vi "Rcv Caller Notice.vi"(7 "Actor Name":string, 8 "error in (no error)":errorcluster, 9 "Params":variant, 10 "Action Name":string, 11 "Generic Actor in":refnum<class "Generic Actor.lvclass">) -> (0 "error out":errorcluster, 3 "Generic Actor out":refnum<class "Generic Actor.lvclass">)   [LabVIEW 2020, in "Generic Actor.lvlib" / "Generic Actor.lvclass"]
uses:
  Generic Actor.lvclass
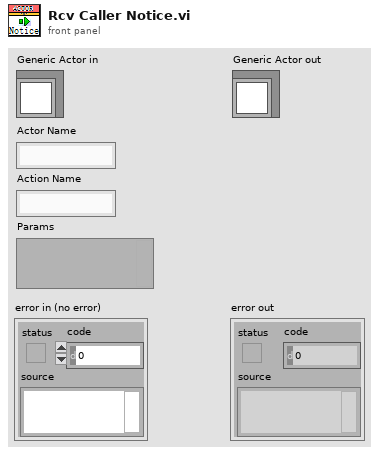
[diagram p1: front panel]
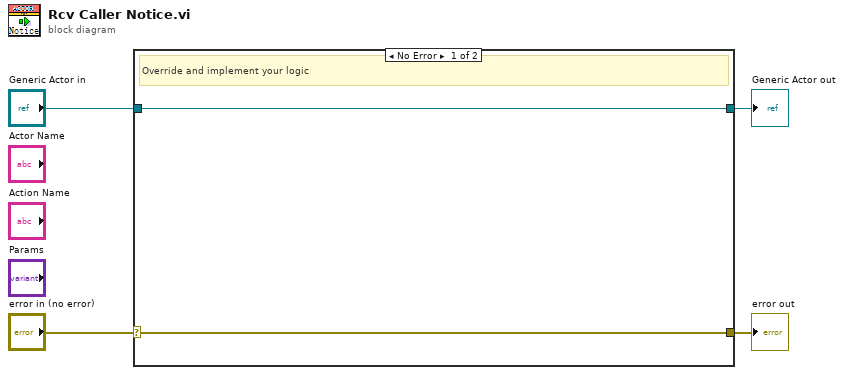
[diagram p0: block diagram]
diagram:
  n1 = case shown="No Error" "error in (no error)" {
    selector: "error in (no error)" -> [w5 w8]
    tunnel: [w5 w8] -> w3
    tunnel: [w6 w7] -> w1
    tunnel: "Generic Actor in" -> [w6 w7]
    frame No Error {
      # "Override and implement your logic"
    }
    frame Error {
    }
  }
  "error out" <- w3
  "Generic Actor out" <- w1
